vi "I2C Loop.vi"   [LabVIEW 2016]
uses:
  Robot Global Data.vi
types:
  T1 = typedef "Drivetrain Command Cluster.ctl" = cluster{"Drivetrain Mode":T2, "Heading Target":dbl, "Turn Power":dbl, "Y Power":dbl, "Center Piston Down?":bool, "Traction?":bool, "Strafe Power":dbl, "Zero Gyro":bool, "Distance Target":dbl, "Strafe Correct":bool, "Y Max Output":dbl, "Y Min Output":dbl, "X Max Output":dbl, "X Min Output":dbl, "Z Max Output":dbl, "Z Min Output":dbl, "Z Target":dbl}
  T2 = typedef "Drivetrain Mode.ctl" = enum16{"Manual", "Gyro Steer", "Distance Drive", "Translate Drive", "PID Drive"}
  T3 = typedef "Intake Control Cluster.ctl" = cluster{"Intake Modes":T4, "Override IR":bool, "Intake Auto States":T5}
  T4 = typedef "Intake Modes.ctl" = enum16{"Manual", "Auto"}
  T5 = typedef "Intake Auto States.ctl" = enum16{"Idle", "Load Ball", "Load Gear", "Outake Gear", "Outake Ball"}
  T6 = typedef "WPI_DriverStationRobotMode2.ctl" = enum16{"Autonomous Disabled", "Autonomous Enabled", "Teleop Disabled", "Teleop Enabled", "Disconnected", "Finish", "Test Disabled", "Test Enabled", "Emergency Stopped"}
  T7 = typedef "WPI_DigitalOutputDevRef.ctl" = cluster{"DIO Channel":T8, "DevStatus":errorcluster}
  T8 = typedef "FPGA_DIOChannel.ctl" = enum8{"DIO 0", "DIO 1", "DIO 2", "DIO 3", "DIO 4", "DIO 5", "DIO 6", "DIO 7", "DIO 8", "DIO 9", "DIO MXP 0", "DIO MXP 1", "DIO MXP 2", "DIO MXP 3", "DIO MXP 4", "DIO MXP 5", "DIO MXP 6", "DIO MXP 7", "DIO MXP 8", "DIO MXP 9", "DIO MXP 10", "DIO MXP 11", "DIO MXP 12", "DIO MXP 13", "DIO MXP 14", "DIO MXP 15", "SPI Port CS1", "SPI Port CS2", "SPI Port CS3", "SPI Port MISO", "SPI Port MOSI", "Invalid"}
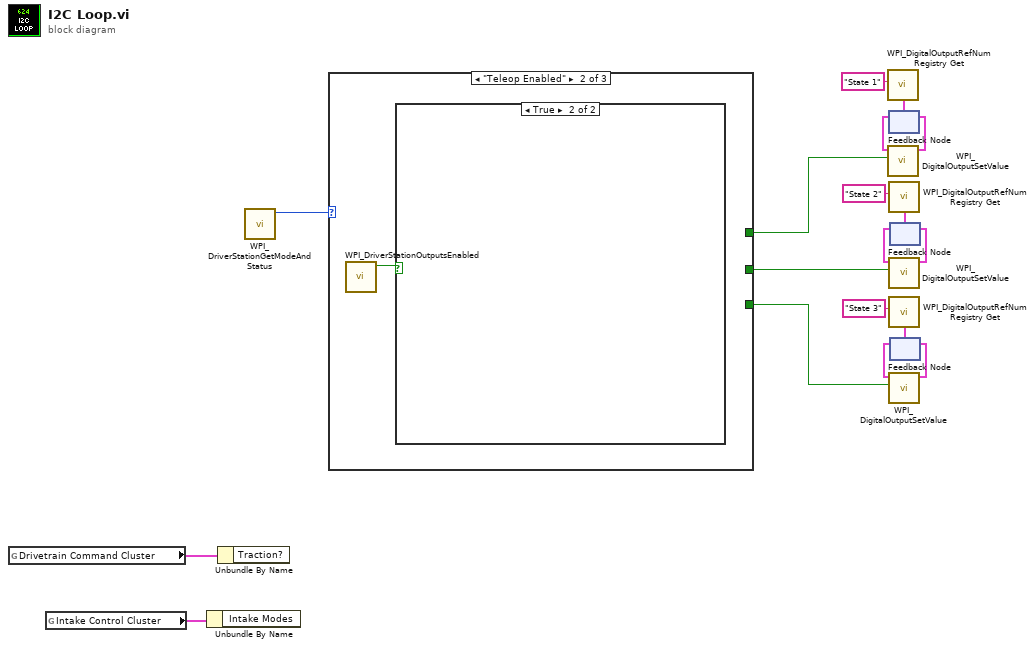
[diagram p0: block diagram]
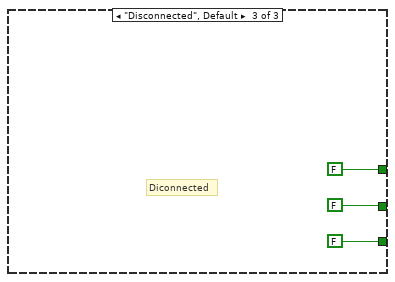
[diagram p4: hidden frame]
diagram:
  n1 = global read "Robot Global Data.vi" "Drivetrain Command Cluster"() -> (w2:T1)
  n2 = global read "Robot Global Data.vi" "Intake Control Cluster"() -> (w1:T3)
  n3 = Unbundle By Name(w1) -> ()  [unwired: 1 out]
  n4 = Unbundle By Name(w2) -> ()  [unwired: 1 out]
  n5 = call <vilib>:"WPI_DriverStationGetModeAndStatus.vi"() -> ("Robot Mode"=w18:T6)  [unwired: 10 in, 1 out]
  n6 = case shown="\"Teleop Enabled\"" w18 {
    tunnel: [_ _ FALSE] -> w3
    tunnel: [_ _ FALSE] -> w4
    tunnel: [_ _ FALSE] -> w5
    frame "Autonomous Enabled" {
      # "Auto"
    }
    frame "Teleop Enabled" {
      n7 = call <vilib>:"WPI_DriverStationOutputsEnabled.vi"() -> ("OutputsEnabled?"=w19:bool)  [unwired: 10 in, 1 out]
      n8 = case shown="True" w19 {
        frame False {
          # "Lost Comm."
        }
        frame True {
        }
      }
    }
    frame "Disconnected", Default {
      # "Diconnected"
    }
  }
  n9 = call <vilib>:"WPI_DigitalOutputRefNum Registry Get.vi"("refnum name"="State 1") -> ("DigitalOutputDevRef"=w15:T7)  [unwired: 9 in, 1 out]
  n10 = feedback #1(w15) -> (w16:T7)
  n11 = call <vilib>:"WPI_DigitalOutputSetValue.vi"("Value"=w3, "DigitalOutputDevRef"=w16) -> ("DigitalOutputDevRef"=w17:T7)  [unwired: 8 in, 1 out]
  n12 = feedback-in #1(w17) -> ()
  n13 = call <vilib>:"WPI_DigitalOutputRefNum Registry Get.vi"("refnum name"="State 2") -> ("DigitalOutputDevRef"=w12:T7)  [unwired: 9 in, 1 out]
  n14 = call <vilib>:"WPI_DigitalOutputRefNum Registry Get.vi"("refnum name"="State 3") -> ("DigitalOutputDevRef"=w7:T7)  [unwired: 9 in, 1 out]
  n15 = feedback #2(w12) -> (w11:T7)
  n16 = call <vilib>:"WPI_DigitalOutputSetValue.vi"("Value"=w4, "DigitalOutputDevRef"=w11) -> ("DigitalOutputDevRef"=w10:T7)  [unwired: 8 in, 1 out]
  n17 = feedback-in #2(w10) -> ()
  n18 = feedback #3(w7) -> (w8:T7)
  n19 = call <vilib>:"WPI_DigitalOutputSetValue.vi"("Value"=w5, "DigitalOutputDevRef"=w8) -> ("DigitalOutputDevRef"=w9:T7)  [unwired: 8 in, 1 out]
  n20 = feedback-in #3(w9) -> ()
